vi "Get density multi sample PN.vi"(3 "N samples":i32=20, 4 "Counter":tag="Dev1/ctr0", 5 "Timing SW trigger":tag="Dev1/port2/line7", 6 "Device":tag="Dev1") -> (0 "Error":errorcluster, 1 "Sample DateTime":timestamp[](array[timestamp]), 2 "Density (kg/m^3)":dbl[](array[numeric]))   [LabVIEW 2010]
uses:
  <vilib>/Platform/TimedLoop/XDataNode/XDataNode.xnode
  <vilib>/Platform/TimedLoop/XDataNode/timing_clust.ctl
  <vilib>/Platform/TimedLoop/XDataNode/nitl_modes.ctl
  <vilib>/Platform/TimedLoop/XDataNode/wakeup.ctl
  <vilib>/DAQmx/read.llb/DAQmx Read (Digital Bool 1Line 1Point).vi
  <vilib>/DAQmx/read.llb/DAQmx Read (Counter U32 1Chan 1Samp).vi
  <vilib>/DAQmx/create/channels.llb/DAQmx Create Channel (CI-Count Edges).vi
  <vilib>/DAQmx/create/channels.llb/DAQmx Create Channel (DI-Digital Input).vi
  <vilib>/daqmx/miscellaneous.llb/DAQmx Fill In Error Info.vi
  <vilib>/Platform/TimedLoop/XDataNode/XDNodeRunTimeDep.lvlib
panel:
  out "current sample":i32
  out "Density history":u32(graph)=997
  in  "stop":bool
  out "reset state":bool
  # "by Paul Nathan, 29/01/2012"
  # "Revisions:\nDate       Desc.      Auth.\nx               x               x"
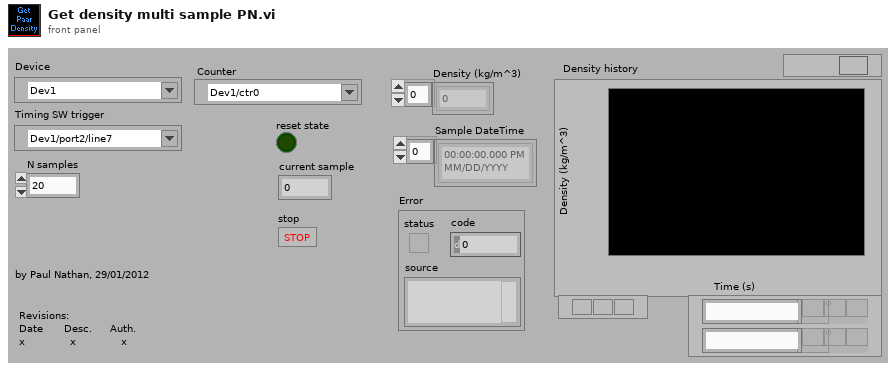
[diagram p1: front panel]
types:
  T1 = typedef "XDNodeRunTimeDep.lvlib/timing_clust.ctl" = cluster{"Expected End [f-1]":u64, "Actual End [f-1]":u64, "Finished Late? [f-1]":bool, "Expected End [i-1]":u64, "Actual End [i-1]":u64, "Finished Late? [i-1]":bool, "Expected Start [i]":u64, "Actual Start [i]":u64, "Expected Start [f]":u64, "Actual Start [f]":u64, "Source Name":string, "Structure Name":string, "Period":i64, "Deadline":i64, "Offset":i64, "Start":i64, "Priority":i32, "Timeout":i32, "Mode":T2, "Wakeup Reason":T3, "Error":errorcluster, "Source Type":string, "Secondary Source Type":string, "Global End Time":u64, "Global Start Time":u64, "Frame Duration":u64, "Iteration Duration":u64, "Assigned CPU":i32, "I/O Scan Engine Mode":u32}
  T2 = typedef "XDNodeRunTimeDep.lvlib/nitl_modes.ctl" = enum32{"No Change", "Process missed periods, maintain original phase", "Discard missed periods, maintain original phase", "Process missed periods, ignore original phase", "Discard missed periods, ignore original phase"}
  T3 = typedef "XDNodeRunTimeDep.lvlib/wakeup.ctl" = enum32{"Normal", "Aborted", "Asynchronous wakeup", "Timing source error", "Timed loop error", "Timeout"}
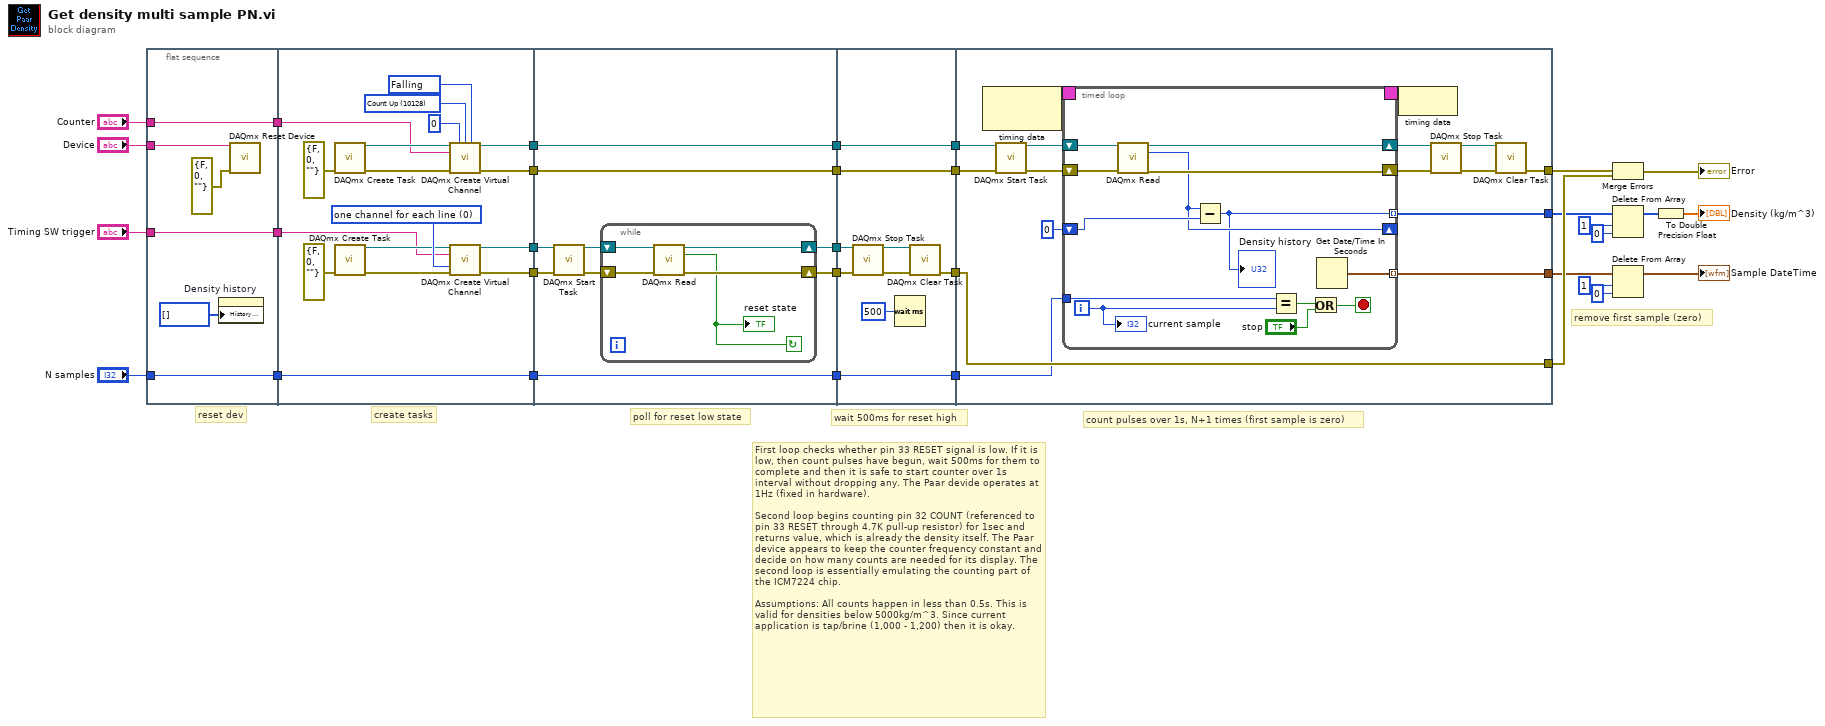
[diagram p0: block diagram]
diagram:
  # "remove first sample (zero)"
  # "count pulses over 1s, N+1 times (first sample is zero)"
  # "wait 500ms for reset high"
  # "poll for reset low state"
  # "create tasks"
  # "reset dev"
  # "First loop checks whether pin 33 RESET signal is low. If it is low, then count pulses have begun, wait 500ms for them to complete and then it is safe to start counter over 1s interval without dropping any. The Paar devide operates at 1Hz (fixed in hardware).\n\nSecond loop begins counting pin 32 COUNT (referenced to pin 33 RESET through 4.7K pull-up resistor) for 1sec and returns value, which is already the density itself. The Paar device appears to keep the counter frequency constant and decide on how many counts are needed for its display. The second loop is essentially emulating the counting part of the ICM7224 chip.\n\nAssumptions: All counts happen in less than 0.5s. This is valid for densities below 5000kg/m^3. Since current application is tap/brine (1,000 - 1,200) then it is okay."
  n1 = flat-sequence {
    tunnel: [w38] -> w30
    tunnel: "Timing SW trigger" -> [w38]
    tunnel: [w37] -> w28
    tunnel: "Counter" -> [w37]
    tunnel: "Device" -> [w36]
    tunnel: [w35] -> w16
    tunnel: "N samples" -> [w35]
    tunnel: w30 -> [w48]
    tunnel: w28 -> [w47]
    tunnel: [w43] -> w24
    tunnel: [w44] -> w22
    tunnel: w16 -> [w42]
    tunnel: [w42] -> w12
    tunnel: [w41] -> w2
    tunnel: [w40] -> w1
    tunnel: [w65] -> w33
    tunnel: [w64] -> w32
    tunnel: [w63] -> w25
    tunnel: w24 -> [w63]
    tunnel: [w62] -> w23
    tunnel: w22 -> [w62]
    tunnel: [w61] -> w13
    tunnel: w12 -> [w61]
    tunnel: w2 -> [w58]
    tunnel: w1 -> [w57]
    tunnel: w33 -> [w76]
    tunnel: w32 -> [w75]
    tunnel: [w74] -> w31
    tunnel: w25 -> [w73]
    tunnel: w23 -> [w72]
    tunnel: [w73] -> w21
    tunnel: [w72] -> w20
    tunnel: [w71] -> w14
    tunnel: w13 -> [w71]
    tunnel: w31 -> [w88]
    tunnel: w21 -> [w86]
    tunnel: w20 -> [w84]
    tunnel: [w89] -> w19
    tunnel: [w88] -> w18
    tunnel: [w87] -> w6
    tunnel: w14 -> [w82]
    tunnel: [w81] -> w4
    frame #0 {
      n2 = property on="Density history" class="WFChart (strict)"("History Data"=u32[] []) -> ()  [unwired: 2 in, 2 out]
      n3 = call <vilib>:"DAQmx Reset Device.vi"("device in"=w36, "error in"=errorcluster {"status"=FALSE, "code"=0, "source"=""}) -> ()  [unwired: 13 in, 1 out]
    }
    frame #1 {
      w52 = 10171 items=["Rising"=10280, "Falling"=10171] ("edge")
      w53 = 10128 items=["Count Up"=10128, "Count Down"=10124, "Externally Controlled"=10326] ("count direction")
      w50 = 0 items=["one channel for each line", "one channel for all lines"] ("line grouping")
      n4 = call <vilib>:"DAQmx Create Task.vi"("error in"=errorcluster {"status"=FALSE, "code"=0, "source"=""}) -> ("task out"=w55:refnum<k21>, "error out"=w56:errorcluster)  [unwired: 13 in]
      n5 = call <vilib>:"DAQmx Create Task.vi"("error in"=errorcluster {"status"=FALSE, "code"=0, "source"=""}) -> ("task out"=w49:refnum<k21>, "error out"=w51:errorcluster)  [unwired: 13 in]
      n6 = call-poly <vilib>:"DAQmx Create Virtual Channel.vi"("task in"=w55, "initial count"=u32 0, "count direction"=w53, "edge"=w52, "counter"=w47, "error in"=w56) -> ("task out"=w44:refnum<k21>, "error out"=w43:errorcluster)  [unwired: 8 in]
      n7 = call-poly <vilib>:"DAQmx Create Virtual Channel.vi"("task in"=w49, "lines"=w48, "line grouping"=w50, "error in"=w51) -> ("task out"=w40:refnum<k21>, "error out"=w41:errorcluster)  [unwired: 10 in]
    }
    frame #2 {
      n8 = call <vilib>:"DAQmx Start Task.vi"("task/channels in"=w57, "error in"=w58) -> ("task out"=w60:refnum<k21>, "error out"=w59:errorcluster)  [unwired: 12 in]
      n9 = while {
        shift-right: [w69] -> w64
        shift-left: w59 -> [w68]
        shift-right: [w67] -> w65
        shift-left: w60 -> [w70]
        stop <- w66 continue-if-true
        n10 = call-poly <vilib>:"DAQmx Read.vi"("task/channels in"=w70, "error in"=w68) -> ("task out"=w67:refnum<k21>, "data"=w66:bool, "error out"=w69:errorcluster)  [unwired: 11 in]
        "reset state" <- w66
      }
    }
    frame #3 {
      n11 = call <vilib>:"DAQmx Stop Task.vi"("task/channels in"=w76, "error in"=w75) -> ("task out"=w77:refnum<k21>, "error out"=w78:errorcluster)  [unwired: 12 in]
      n12 = Wait (ms)(milliseconds to wait=u32 500) -> ()  [unwired: 1 out]
      n13 = call <vilib>:"DAQmx Clear Task.vi"("task in"=w77, "error in"=w78) -> ("error out"=w74:errorcluster)  [unwired: 13 in]
    }
    frame #4 {
      n14 = node-c288() -> (w95:T1)  [unwired: 1 in]
      n15 = call <vilib>:"DAQmx Start Task.vi"("task/channels in"=w84, "error in"=w86) -> ("task out"=w83:refnum<k21>, "error out"=w85:errorcluster)  [unwired: 12 in]
      n16 = timed-loop {
        tunnel: [w96] -> w87 mode=indexing
        shift-right: [w106] -> w91
        shift-left: w83 -> [w107]
        shift-right: [w105] -> w90
        shift-left: w85 -> [w108]
        timing: w95 -> [_]
        timing-out: [_] -> w94
        tunnel: w82 -> [w104]
        tunnel: [w103] -> w81 mode=indexing
        shift-right: [w97] -> _
        shift-left: u32 0 ("data") -> [w98]
        i -> [w102]
        stop <- w100 stop-if-true
        n17 = call-poly <vilib>:"DAQmx Read.vi"("task/channels in"=w107, "error in"=w108) -> ("task out"=w106:refnum<k21>, "data"=w97:u32, "error out"=w105:errorcluster)  [unwired: 11 in]
        n18 = Subtract(x=w97, y=w98) -> (x-y=w96:u32)
        "Density history" <- w96
        n19 = Equal?(x=w104, y=w102) -> (x = y?=w101:bool)
        n20 = Or(x=w101, y="stop") -> (x .or. y?=w100:bool)
        n21 = Get Date/Time In Seconds() -> (seconds since 1Jan1904=w103:timestamp)
        "current sample" <- w102
      }
      n22 = node-c288(w94) -> ()
      n23 = call <vilib>:"DAQmx Stop Task.vi"("task/channels in"=w91, "error in"=w90) -> ("task out"=w92:refnum<k21>, "error out"=w93:errorcluster)  [unwired: 12 in]
      n24 = call <vilib>:"DAQmx Clear Task.vi"("task in"=w92, "error in"=w93) -> ("error out"=w89:errorcluster)  [unwired: 13 in]
    }
  }
  n25 = Merge Errors(w19, w18) -> (→"Error":errorcluster)
  n26 = Delete From Array(array=w6, length=1, index=0) -> (array with subset deleted=w5:u32[])  [unwired: 1 out]
  n27 = Delete From Array(array=w4, length=1, index=0) -> (array with subset deleted=→"Sample DateTime":timestamp[])  [unwired: 1 out]
  n28 = To Double Precision Float(number=w5) -> (double precision float=→"Density (kg/m^3)":dbl[])
